vi "NF87XX.Drive to Indexmark.vi"(0 "i ref in":refnum<vi>, 1 "System":string="N/A", 2 "Forward?":bool, 5 "error in (no error)":errorcluster) -> (14 "i ref out":refnum<vi>, 19 "error out":errorcluster)   [LabVIEW 2014, in "NF87XX.lvlib"]
doc: "Drives to the limit (endswitch) in specified direction.\n\nauthor: Stefan Götte\ndata: 09-JAN-2007\n\n\nLicense Agreement for this software:\n\nCopyright (C)\nGesellschaft für Schwerionenforschung, GSI\nPlanckstr. 1\n64291 Darmstadt\nGermany\n\nContact: D.Beck@gsi.de \n\nThis program is free software; you can redistribute it and/or modify it under the terms of the GNU General Public License as published by the Free Software Foundation; either version 2 of the license, or (at your option) any later version.\n\nThis program is distributed in the hope that it will be useful, but WITHOUT ANY WARRANTY; without even the implied warranty of MERCHANTABILITY or FITNESS FOR A PARTICULAR PURPOSE. See the GNU General License for more details (http://www.gnu.org).\n\nGesellschaft für Schwerionenforschung, GSI\nPlanckstr. 1, 64291 Darmstadt, Germany\nFor all questions and ideas contact: M.Richter@gsi.de, H.Brand@gsi.de or D.Beck@gsi.de.\nLast update: 17-JUN-2004"
uses:
  NF87XX.lvlib
  non_GPL/instr.lib/NewFocusPico/Pico Parameters.ctl
  non_GPL/instr.lib/NewFocusPico/NewFocusPico - Driver np.lvlib
panel:
  in  "Pico Parameter type":T1={"Pico Type"=enum."Open-Loop Pico", "Acceleration (steps/sec^2)"="32000", "Velocity ( Hz)"="2000", "Driver"="A1", "Motor"="0", "Channel"="0", "Process Step"="Final Test"}
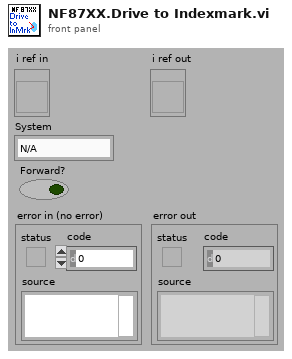
[diagram p1: front panel]
types:
  T1 = typedef "NewFocusPico - Driver np.lvlib/Pico Parameters.ctl" = cluster{"Pico Type":enum16{"Open-Loop Pico", "Close-Loop Pico", "Pico Ultra"}, "Acceleration (steps/sec^2)":string, "Velocity ( Hz)":string, "Driver":string, "Motor":string, "Channel":string, "Process Step":string}
  T2 = enum16{"User....", "DEF", "DIAG", "INI", "LOCK", "UNLOCK", "MAP", "SAV", "VER", "ACC", "CHL", "FOR", "GO", "HAL", "MOF", "MON", "MPV", "POS", "REL", "REV", "STA", "STO", "TYP", "VEL", "ABS", "SER", "NOS", "DRT", "FLI", "RLI", "FIN", "RIN", "AIN", "IN", "JOF", "JON", "OUT", "RES FINE", "RES COARSE", "02 (HEX)", "PWM", "CNT", "TMR", "HOSTNAME", "IPADDR", "IPMODE", "NETMASK", "GATEWAY", "DNSSRVR", "PASSWD", "ECHO", "MACADDR"}
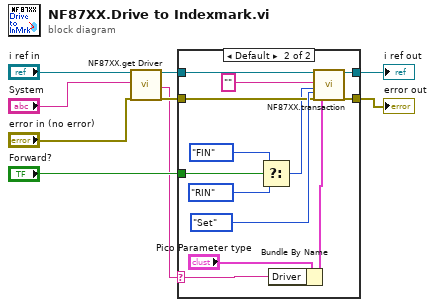
[diagram p0: block diagram]
diagram:
  n1 = call "NF87XX.get Driver.vi"("i ref in"="i ref in", "System"="System", "error in (no error)"="error in (no error)") -> ("i ref out"=w4:refnum<vi>, "Driver"=w1:string, "error out"=w5:errorcluster)  [unwired: 12 in, 2 out]
  n2 = case shown="Default" w1 {
    selector: w1 -> [_ w12]
    tunnel: [w11 w24] -> w9
    tunnel: [w10 w23] -> w8
    tunnel: w5 -> [w10 w20]
    tunnel: w4 -> [w11 w19]
    tunnel: "Forward?" -> [_ w16]
    frame "N/A" {
    }
    frame Default {
      n3 = Select(t=T2."FIN" ("MCL Cmd"), s=w16, f=T2."RIN" ("MCL Cmd")) -> (s? t:f=w13:T2)
      n4 = Bundle By Name(cluster="Pico Parameter type", "Driver"=w12) -> (w17:T1)
      n5 = call "NF87XX.transaction.vi"("i ref in"=w19, "User Cmd/Numeric Argu"="", "MCL Cmd"=w13, "Query/Set"=enum16{"Query", "Set"}."Set", "error in (no error)"=w20, "Pico Parameter"=w17) -> ("i ref out"=w24:refnum<vi>, "error out"=w23:errorcluster)  [unwired: 11 in, 1 out]
    }
  }
  "error out" <- w8
  "i ref out" <- w9
